vi "post_dust_source.vi"(8 "error in (no error)":errorcluster, 11 "Dust control settings":T1={"Integer Timestamp"=8, "Einzel Voltage"=2.0, "Needle Voltage"=3.0, "Frequency"=4.0, "Width (ms) : 0.1 "=5.0, "Desired Amplitude (V)"=6.0, "X Voltage"=7.0, "Y Voltage"=0.0, "Settings ID"="", "ID#"=0} {"Needle Voltage" min=0.0 max=10.0 step=0.01 format="%.2g"; "Y Voltage" min=0.0 max=9.0 step=0.01 format="%.2g"; "X Voltage" min=0.0 max=9.0 step=0.01 format="%.2g"; "Einzel Voltage" min=0.0 max=10.0 step=0.01 format="%.2g"; "Desired Amplitude (V)" min=0.0 max=10.0 step=0.01 format="%5.2f"; "Width (ms) : 0.1" min=0.05 max=5.0 step=0.01 format="%6.2f"; "Frequency" min=1.0 max=100.0 step=0.01 format="%.1f"}) -> (0 "error out":errorcluster)   [LabVIEW 2013]
doc: "Adds a new row to the source_settings table."
uses:
  User Interface/Controls/dust_source_control.ctl
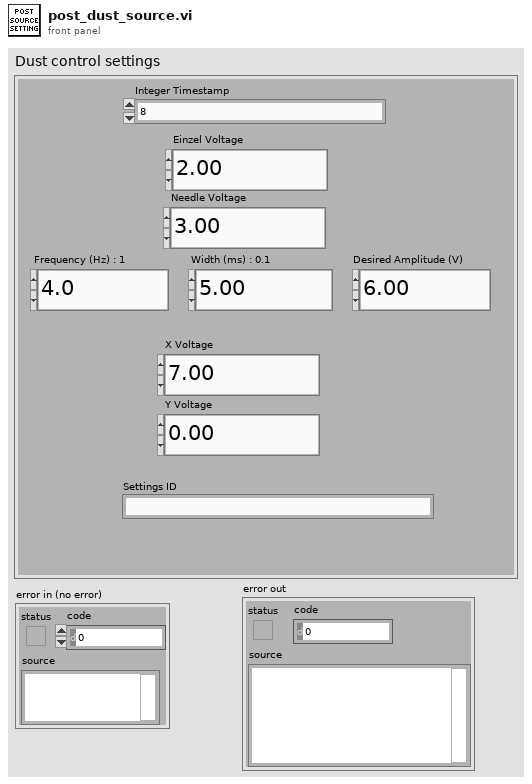
[diagram p1: front panel]
types:
  T1 = typedef "dust_source_control.ctl" = cluster{"Integer Timestamp":u64, "Einzel Voltage":dbl, "Needle Voltage":dbl, "Frequency":dbl, "Width (ms) : 0.1 ":dbl, "Desired Amplitude (V)":dbl, "X Voltage":dbl, "Y Voltage":dbl, "Settings ID":string, "ID#":i32}
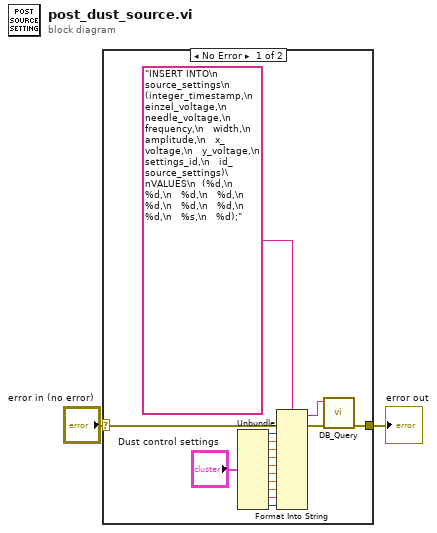
[diagram p0: block diagram]
diagram:
  n1 = case shown="No Error" "error in (no error)" {
    selector: "error in (no error)" -> [w18 w19]
    tunnel: [w12 w19] -> w1
    frame No Error {
      n2 = Unbundle("Dust control settings") -> ("Integer Timestamp"=w15:u64, "Einzel Voltage"=w11:dbl, "Needle Voltage"=w10:dbl, "Frequency"=w9:dbl, "Width (ms) : 0.1"=w8:dbl, "Desired Amplitude (V)"=w7:dbl, "X Voltage"=w6:dbl, "Y Voltage"=w5:dbl, "Settings ID"=w4:string, "ID#"=w3:i32)
      n3 = Format Into String(format string="INSERT INTO\n  source_settings\n  (integer_timestamp,\n   einzel_voltage,\n   needle_voltage,\n   frequency,\n   width,\n   amplitude,\n   x_voltage,\n   y_voltage,\n   settings_id,\n   id_source_settings)\nVALUES\n  (%d,\n   %d,\n   %d,\n   %d,\n   %d,\n   %d,\n   %d,\n   %d,\n   %s,\n   %d);" ("table"), error in=w18, w15, w11, w10, w9, w8, w7, w6, w5, w4, w3) -> (resulting string=w14:string, error out=w17:errorcluster)  [unwired: 1 in]
      n4 = call "DB_Query.vi"("error in (no error)"=w17, "Parameterized Query"=w14) -> ("error out"=w12:errorcluster)  [unwired: 7 in, 2 out]
    }
    frame Error {
    }
  }
  "error out" <- w1
